vi "Write_firstConnection.vi"(8 "error in (no error)":errorcluster, 10 "firstConnection":bool, 11 "TcpServerCmd in":refnum<class "TcpServerCmd.lvclass">) -> (0 "error out":errorcluster, 3 "TcpServerCmd out":refnum<class "TcpServerCmd.lvclass">)   [LabVIEW 2018, in "TcpServerCmd.lvclass"]
doc: "Write firstConnection boolean to know if TCP Client connected to TCP Server at first time or not."
uses:
  TcpServerCmd.lvclass
  TcpServerCmd.lvclass/TcpServerCmd.ctl
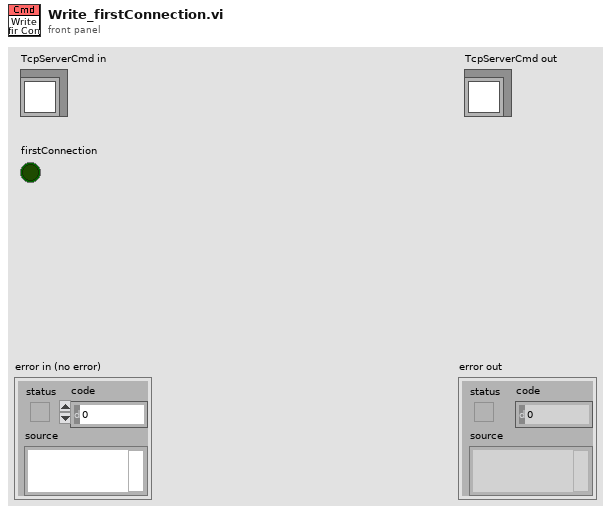
[diagram p1: front panel]
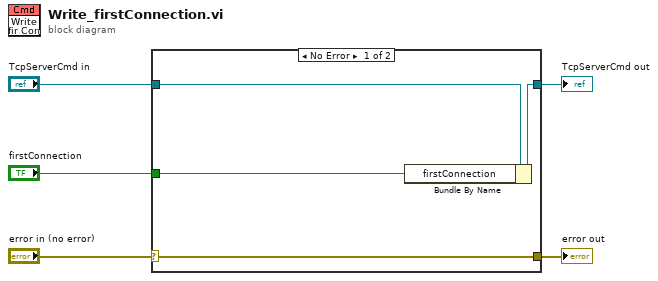
[diagram p0: block diagram]
diagram:
  n1 = case shown="No Error" "error in (no error)" {
    selector: "error in (no error)" -> [w9 w10]
    tunnel: [w9 w10] -> w4
    tunnel: [w7 w11] -> w2
    tunnel: "TcpServerCmd in" -> [w8 w11]
    tunnel: "firstConnection" -> [w6 _]
    frame No Error {
      n2 = Bundle By Name(cluster=w8, "firstConnection"=w6) -> (w7:refnum<class "TcpServerCmd.lvclass">)
    }
    frame Error {
    }
  }
  "error out" <- w4
  "TcpServerCmd out" <- w2
